vi "Get_Relative_VI_Path.vi"(8 "error in (no error)":errorcluster, 11 "UI_Interaction_Manager in":refnum<class "UI_Interaction_Manager.lvclass">) -> (0 "error out":errorcluster, 2 "Relative VI Path":path, 3 "UI_Interaction_Manager out":refnum<class "UI_Interaction_Manager.lvclass">)   [LabVIEW 2011, in "UI_Interaction_Manager.lvclass"]
uses:
  UI_Interaction_Manager.lvclass
  UI_Interaction_Manager.lvclass/UI_Interaction_Manager.ctl
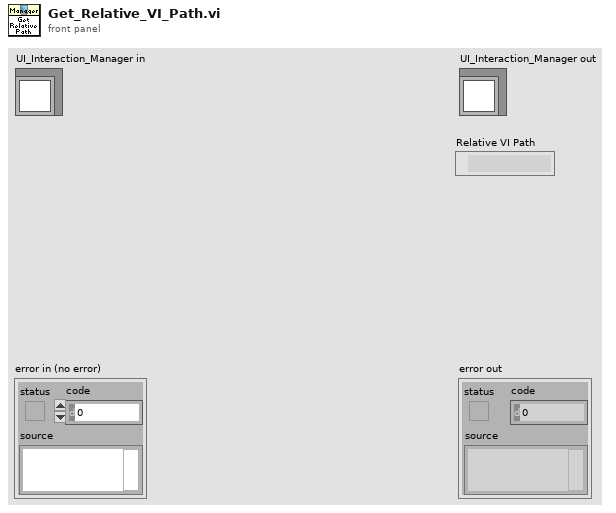
[diagram p1: front panel]
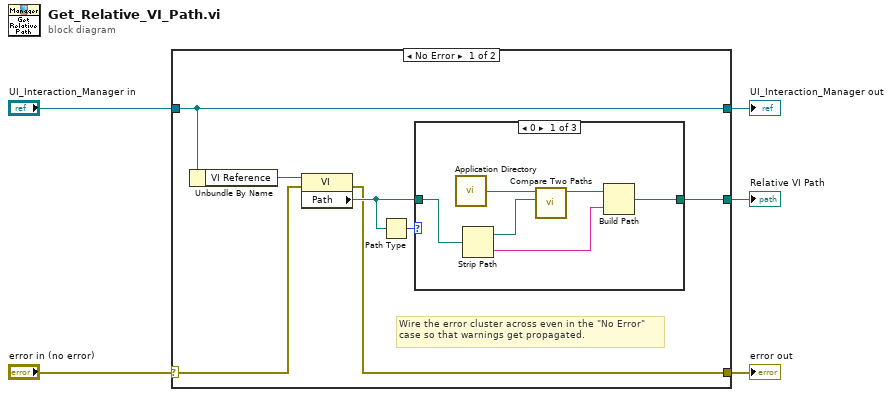
[diagram p0: block diagram]
diagram:
  n1 = case shown="No Error" "error in (no error)" {
    selector: "error in (no error)" -> [w10 w22]
    tunnel: [w6 w22] -> w4
    tunnel: [w12 w21] -> w2
    tunnel: "UI_Interaction_Manager in" -> [w12 w21]
    tunnel: [w7 _] -> w1
    frame No Error {
      # "Wire the error cluster across even in the \"No Error\"\ncase so that warnings get propagated."
      n2 = Unbundle By Name(w12) -> ("VI Reference"=w11:refnum<vi>)
      n3 = property class="VI"(reference=w11, error in=w10) -> (error out=w6:errorcluster, "Path"=w8:path)  [unwired: 1 out]
      n4 = Path Type(1:w8) -> (0:w9:i16)
      n5 = case shown="0" w9 {
        tunnel: w8 -> [w14 w19 w20]
        tunnel: [w13 w19 w20] -> w7
        frame 0 {
          n6 = call <vilib>:"Application Directory.vi"() -> ("Application Directory"=w16:path)
          n7 = Strip Path(path=w14) -> (stripped path=w15:path, name=w17:string)
          n8 = call <vilib>:"Compare Two Paths.vi"("Path 2"=w15, "Path 1"=w16) -> ("Relative Path from 1 to 2"=w18:path)  [unwired: 6 in, 3 out]
          n9 = Build Path(base path=w18, name or relative path=w17) -> (appended path=w13:path)
        }
        frame 1 {
        }
        frame Default {
        }
      }
    }
    frame Error {
    }
  }
  "error out" <- w4
  "UI_Interaction_Manager out" <- w2
  "Relative VI Path" <- w1
